vi "Algorithym in progress.vi"() -> ()   [LabVIEW 2016]
uses:
  Enums/Start position.ctl
panel:
  in  "Start Y 3":dbl
  in  "Start Y 2":dbl
  in  "Start Y 1":dbl
  in  "Hopper Y":dbl
  in  "Hopper X":dbl
  in  "Start X":dbl
  in  "Start":T1
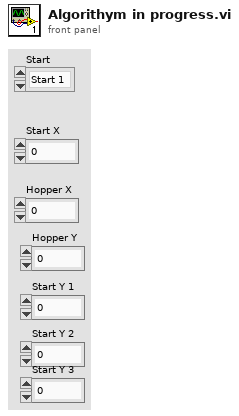
[diagram p1: front panel]
types:
  T1 = typedef "Start position.ctl" = enum16{"Start 1", "Start 2", "Start 3"}
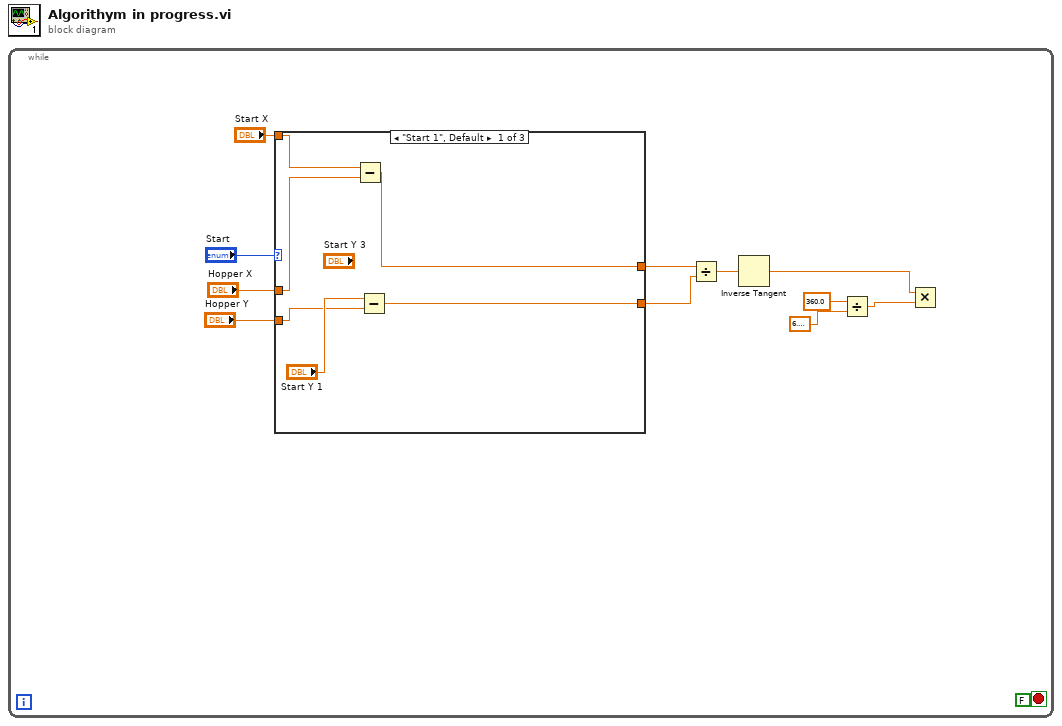
[diagram p0: block diagram]
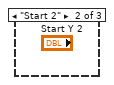
[diagram p2: hidden frame]
diagram:
  n1 = while {
    stop <- FALSE stop-if-true
    n2 = case shown="\"Start 1\", Default" "Start" {
      tunnel: "Start X" -> [w18 _ _]
      tunnel: "Hopper Y" -> [w15 _ _]
      tunnel: "Hopper X" -> [w17 _ _]
      tunnel: [w14 _ _] -> w6
      tunnel: [w13 _ _] -> w5
      frame "Start 1", Default {
        n3 = Subtract(x=w18, y=w17) -> (x-y=w14:dbl)
        n4 = Subtract(x="Start Y 1", y=w15) -> (x-y=w13:dbl)
      }
      frame "Start 2" {
      }
      frame "Start 3" {
      }
    }
    n5 = Divide(x=w6, y=w5) -> (x/y=w7:dbl)
    n6 = Inverse Tangent(1:w7) -> (0:w1:dbl)
    n7 = Divide(x=360.0, y=6.283185307179586) -> (x/y=w2:dbl)
    n8 = Multiply(x=w1, y=w2) -> ()  [unwired: 1 out]
  }
